vi "New Express VI.vi"(8 "error in (no error)":errorcluster, 10 "App Refnum":refnum<vi>, 11 "SubVI Refnum":refnum<vi>) -> (0 "error out":errorcluster, 3 "Express VI Type out":refnum<class "Express VI Type.lvclass">)   [LabVIEW 2020, in "Peek Window.lvlib" / "Express VI Type.lvclass"]
uses:
  Express VI Type.lvclass
  D:/Code/VI-Peek/source/Peek Window/VI Types/Standard VI Type/Standard VI Type.lvclass
  Implementation VI Type/Implementation VI Type.lvclass
  Standard VI Type/Standard VI Type.lvclass/Standard VI Type.ctl
  Express VI Type.lvclass/Express VI Type.ctl
  Standard VI Type/Write App Refnum.vi
  Standard VI Type/Write Openable.vi
  Standard VI Type/Write Selectable.vi
  Standard VI Type/Write Full Qualified Name.vi
  Standard VI Type/Write VI Refnum.vi
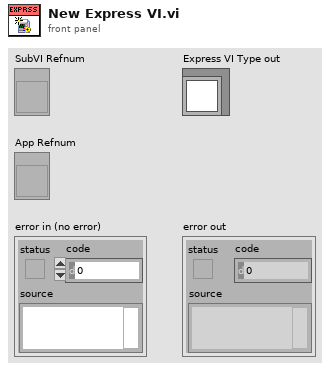
[diagram p1: front panel]
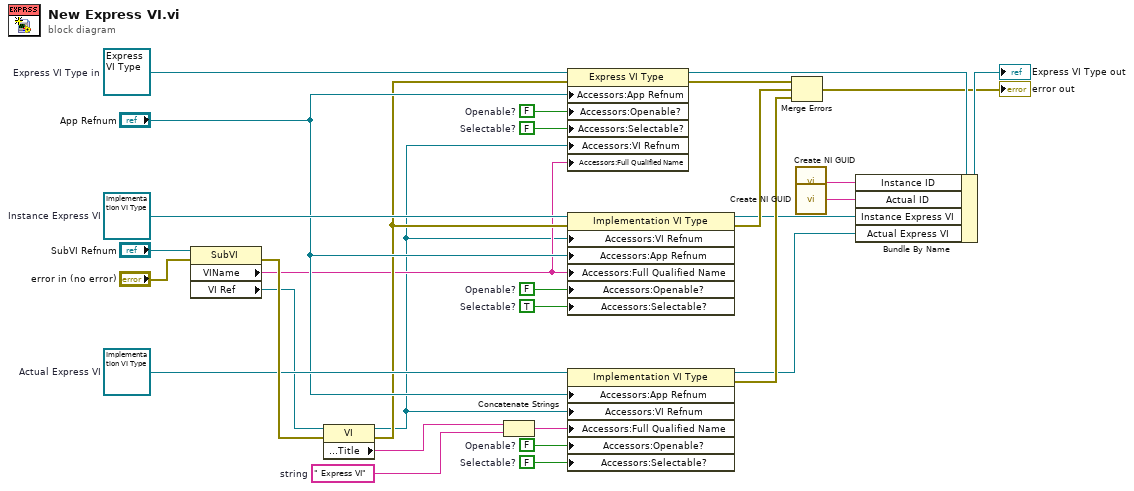
[diagram p0: block diagram]
diagram:
  w14 = TRUE  # Selectable?
  w15 = FALSE  # Openable?
  w16 = FALSE  # Selectable?
  w17 = FALSE  # Openable?
  w18 = FALSE  # Selectable?
  w19 = refnum<class "Implementation VI Type.lvclass"> refnum  # Actual Express VI
  w23 = " Express VI"  # string
  w26 = FALSE  # Openable?
  w28 = refnum<class "Implementation VI Type.lvclass"> refnum  # Instance Express VI
  w30 = refnum<class "Express VI Type.lvclass"> refnum  # Express VI Type in
  n1 = property class="SubVI"(reference="SubVI Refnum", error in="error in (no error)") -> (error out=w27:errorcluster, "VIName"=w2:string, "VI Ref"=w4:refnum<vi>)  [unwired: 1 out]
  n2 = property class="VI"(reference=w4, error in=w27) -> (reference out=w1:refnum<vi>, error out=w10:errorcluster, "Front Panel.Title"=w22:string)
  n3 = Concatenate Strings(w22, w23) -> (w3:string)
  n4 = property class="Express VI Type"(reference=w30, error in=w10, "Accessors:App Refnum"="App Refnum", "Accessors:Openable?"=w26, "Accessors:Selectable?"=w18, "Accessors:VI Refnum"=w1, "Accessors:Full Qualified Name"=w2) -> (reference out=w21:refnum<class "Express VI Type.lvclass">, error out=w24:errorcluster)
  n5 = property class="Implementation VI Type"(reference=w28, error in=w10, "Accessors:VI Refnum"=w1, "Accessors:App Refnum"="App Refnum", "Accessors:Full Qualified Name"=w2, "Accessors:Openable?"=w15, "Accessors:Selectable?"=w14) -> (reference out=w6:refnum<class "Implementation VI Type.lvclass">, error out=w8:errorcluster)
  n6 = property class="Implementation VI Type"(reference=w19, "Accessors:App Refnum"="App Refnum", "Accessors:VI Refnum"=w1, "Accessors:Full Qualified Name"=w3, "Accessors:Openable?"=w17, "Accessors:Selectable?"=w16) -> (reference out=w5:refnum<class "Implementation VI Type.lvclass">, error out=w7:errorcluster)  [unwired: 1 in]
  n7 = Merge Errors(w24, w8, w7) -> (→"error out":errorcluster)
  n8 = call <vilib>:"Create NI GUID.vi"() -> ("NI GUID"=w12:string)
  n9 = call <vilib>:"Create NI GUID.vi"() -> ("NI GUID"=w11:string)
  n10 = Bundle By Name(cluster=w21, "Instance ID"=w12, "Actual ID"=w11, "Instance Express VI"=w6, "Actual Express VI"=w5) -> (→"Express VI Type out":refnum<class "Express VI Type.lvclass">)
